vi "ExpandDir.vi"(11 "Atom In":refnum<class "Atom.lvclass">) -> (1 "InwardDir":T1, 3 "OutwardDir":T1)   [LabVIEW 2020, in "Atom.lvclass"]
uses:
  Atom.lvclass
  Type Defs/Direction Enum.ctl
  Atom.lvclass/Atom.ctl
  Type Defs/SB Type Defs.lvlib
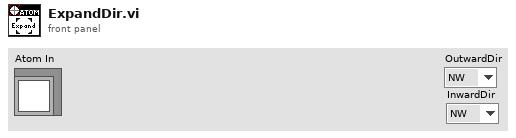
[diagram p1: front panel]
types:
  T1 = typedef "SB Type Defs.lvlib/Direction Enum.ctl" = enum16{"NW", "N", "NE", "E", "SE", "S", "SW", "W"}
  T2 = typedef "Common.lvlib/Position.ctl" = cluster{"Column":i32, "Row":i32}
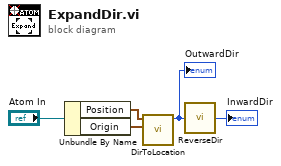
[diagram p0: block diagram]
diagram:
  n1 = Unbundle By Name("Atom In") -> ("Position"=w2:T2, "Origin"=w1:T2)
  n2 = call "DirToLocation.vi"("Origin"=w1, "Position"=w2) -> ("Direction"=w4:T1)  [unwired: 9 in]
  "OutwardDir" <- w4
  n3 = call "ReverseDir.vi"("Direction"=w4) -> ("Direction Out"=→"InwardDir":T1)
